vi "PH_ImageOperator.evt call set Center.vi"(0 "i ref in":refnum<vi>, 1 "Instance":string, 5 "error in (no error)":errorcluster) -> (14 "i ref out":refnum<vi>, 19 "error out":errorcluster)   [LabVIEW 2014, in "PH_ImageOperator.lvlib"]
doc: "This VI calls the event case \"SetCenter\" by a simple call."
uses:
  PH_ImageOperator.lvlib
  CS_Core/BaseProcess/BaseProcess.lvlib
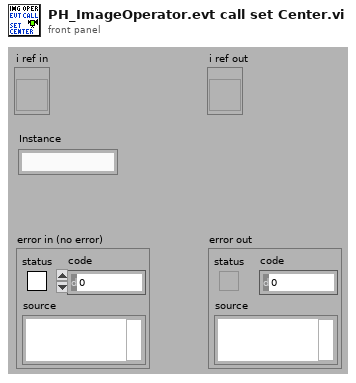
[diagram p1: front panel]
types:
  T1 = enum16{"simple", "synchronous", "asynchronous", "notification"}
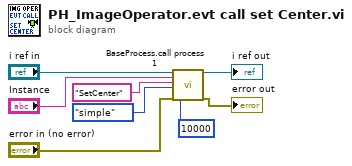
[diagram p0: block diagram]
diagram:
  n1 = call "BaseProcess.call process 1.vi"("i ref in"="i ref in", "Object"="Instance", "Selector"="SetCenter", "CallType"=T1."simple", "error in (no error)"="error in (no error)", "timeout (ms)"=10000) -> ("i ref out"=→"i ref out":refnum<vi>, "error out"=→"error out":errorcluster)  [unwired: 11 in, 1 out]
